vi "Agilent34410A VisaRW.vi"(0 "VISA Rsrc":refnum<visa-resource-name>="SR530", 1 "Timeout ms":u32=1000, 2 "EOS (Aucun)":string, 3 "Délais (0 ms)":u32, 5 "ChaineCom":string caption="Chaîne de commande", 7 "Nbcomm":i32=1 caption="Nombre de \nCommandes", 9 "Nbcaract":u32=100 caption="Nombre de \ncaractères à lire", 11 "error in (no error)":errorcluster, 12 "Lecture?(T)":bool=TRUE, 13 "Poll?(F)":bool) -> (4 "VISA Rsrc Out":refnum<visa-resource-name>="GPIB0::12::INSTR", 6 "ChaineRep":string caption="Chaîne de réponse", 8 "octet d'état":u16, 14 "Count out":u32=44 caption="Nombre de caractères lus", 15 "error out":errorcluster)   [LabVIEW 2019]
doc: "Ce VI envoie des commande d'écriture et de lecture VISA à l'appareil GPIB. Il permet de ne pas séparer un question de sa réponse. Pour que cela fonctionne toute lecture d'un instrument doit se faire par ce VI."
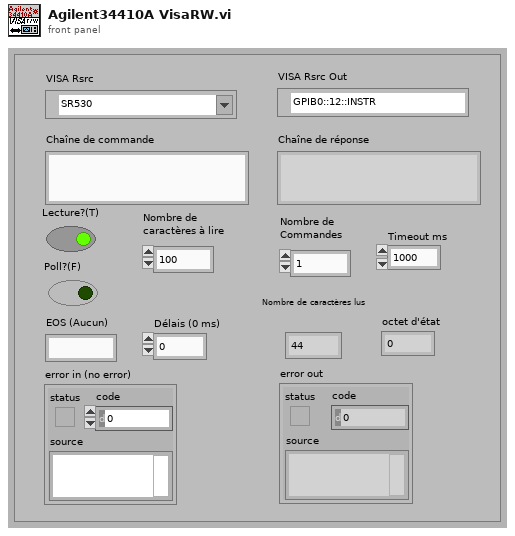
[diagram p1: front panel]
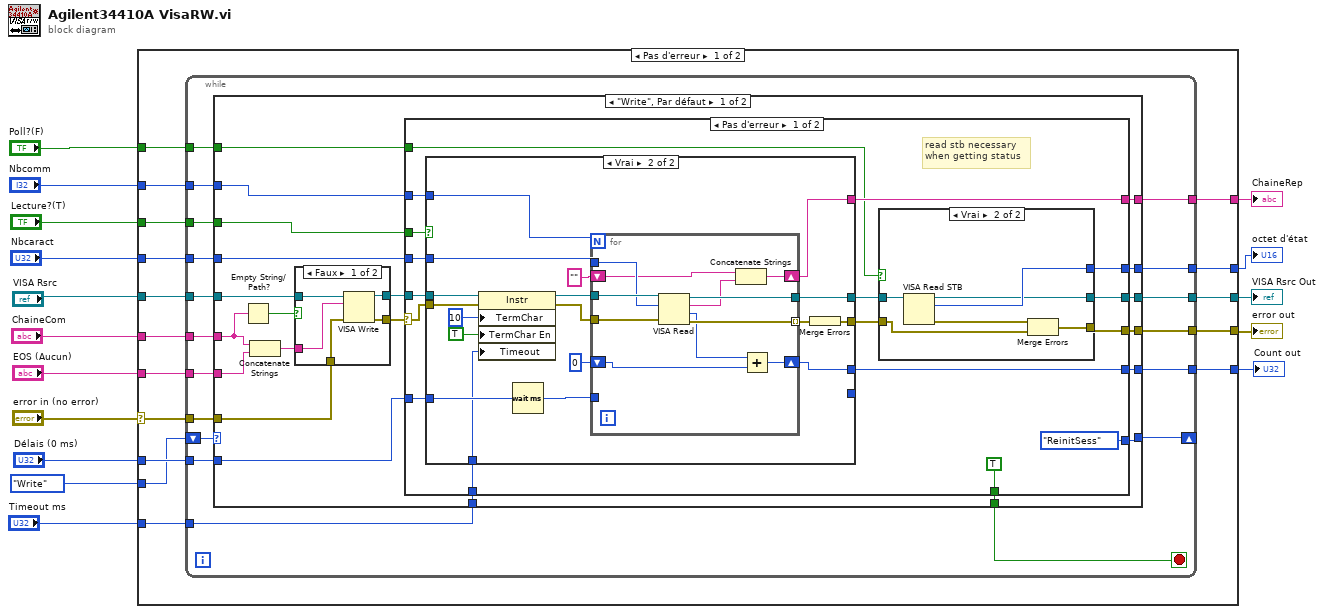
[diagram p0: block diagram]
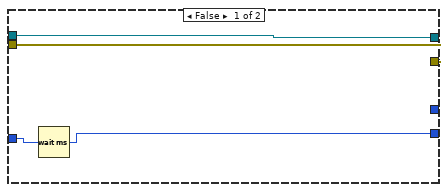
[diagram p3: hidden frame]
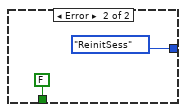
[diagram p4: hidden frame]
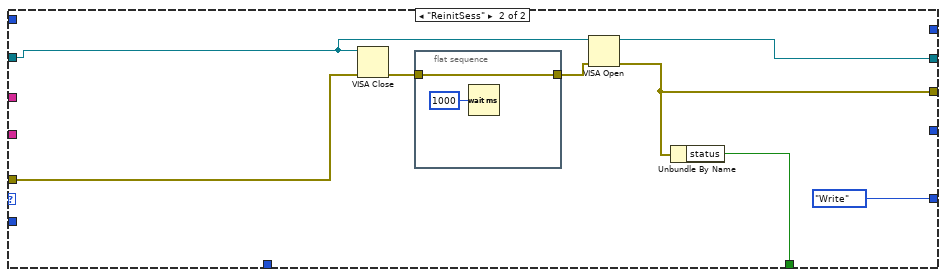
[diagram p6: hidden frame]
diagram:
  n1 = case shown="Pas d'erreur" "error in (no error)" {
    selector: "error in (no error)" -> [w30 w150]
    tunnel: "VISA Rsrc" -> [w31 w149]
    tunnel: [w21 w149] -> w9
    tunnel: "ChaineCom" -> [w23 _]
    tunnel: "EOS (Aucun)" -> [w32 _]
    tunnel: "Délais (0 ms)" -> [w29 _]
    tunnel: "Nbcaract" -> [w28 _]
    tunnel: "Lecture?(T)" -> [w27 _]
    tunnel: [w20 w150] -> w11
    tunnel: "Nbcomm" -> [w24 _]
    tunnel: [w26 _] -> w7
    tunnel: [w25 _] -> w6
    tunnel: "Poll?(F)" -> [w22 _]
    tunnel: [w19 _] -> w3
    tunnel: enum16{"Write", "ReinitSess"}."Write" -> [w18 _]
    tunnel: "Timeout ms" -> [w17 _]
    frame No Error {
      n2 = while {
        tunnel: w32 -> [w50]
        tunnel: w31 -> [w49]
        tunnel: w30 -> [w48]
        tunnel: w29 -> [w47]
        tunnel: w28 -> [w46]
        tunnel: w27 -> [w45]
        tunnel: [w44] -> w26
        tunnel: [w43] -> w25
        tunnel: w24 -> [w42]
        tunnel: w23 -> [w41]
        tunnel: w22 -> [w40]
        tunnel: [w39] -> w21
        tunnel: [w38] -> w20
        tunnel: [w37] -> w19
        shift-right: [w35] -> _
        shift-left: w18 -> [w36]
        tunnel: w17 -> [w33]
        stop <- w34 stop-if-true
        n3 = case shown="\"Write\", Par défaut" w36 {
          tunnel: w50 -> [w71 _]
          tunnel: w49 -> [w69 w145]
          tunnel: w48 -> [w68 w146]
          tunnel: w47 -> [w66 _]
          tunnel: w46 -> [w65 _]
          tunnel: w45 -> [w64 _]
          tunnel: [w63 _] -> w44
          tunnel: [w62 _] -> w43
          tunnel: w42 -> [w61 _]
          tunnel: w41 -> [w60 _]
          tunnel: w40 -> [w58 _]
          tunnel: [w57 w144] -> w39
          tunnel: [w56 w142] -> w38
          tunnel: [w55 _] -> w37
          tunnel: [w54 enum16{"Write", "ReinitSess"}."Write"] -> w35
          tunnel: [w52 w141] -> w34
          tunnel: w33 -> [w51 _]
          frame "Write", Default {
            n4 = Empty String/Path?(string/path=w60) -> (empty?=w59:bool)
            n5 = Concatenate Strings(w60, w71) -> (w70:string)
            n6 = case shown="Faux" w59 {
              tunnel: w70 -> [w136 _]
              tunnel: w69 -> [w135 w138]
              tunnel: w68 -> [w134 w137]
              tunnel: [w133 w138] -> w67
              tunnel: [w132 w137] -> w53
              frame False {
                n7 = VISA Write(VISA resource name=w135, write buffer=w136, error in (no error)=w134) -> (VISA resource name out=w133:refnum<visa-resource-name>, error out=w132:errorcluster)  [unwired: 1 out]
              }
              frame True {
              }
            }
            n8 = case shown="Pas d'erreur" w53 {
              selector: w53 -> [w74 _]
              tunnel: w67 -> [w88 _]
              tunnel: w66 -> [w87 _]
              tunnel: w65 -> [w86 _]
              tunnel: w64 -> [w85 _]
              tunnel: [w84 _] -> w63
              tunnel: [w83 _] -> w62
              tunnel: w61 -> [w82 _]
              tunnel: w58 -> [w81 _]
              tunnel: [w78 _] -> w57
              tunnel: [w77 _] -> w56
              tunnel: [w76 _] -> w55
              tunnel: [enum16{"Write", "ReinitSess"}."ReinitSess" enum16{"Write", "ReinitSess"}."ReinitSess"] -> w54
              tunnel: [TRUE FALSE] -> w52
              tunnel: w51 -> [w72 _]
              frame No Error {
                # "read stb necessary\nwhen getting status"
                n9 = case shown="Vrai" w85 {
                  tunnel: w88 -> [w100 w118]
                  tunnel: [w100 w103] -> w79
                  tunnel: w74 -> [w99 w107]
                  tunnel: [w99 w102] -> w80
                  tunnel: w86 -> [_ w116]
                  tunnel: w87 -> [w98 w115]
                  tunnel: w82 -> [_ w109]
                  tunnel: [_ w111] -> w84
                  tunnel: [_ w110] -> w83
                  tunnel: w72 -> [_ w101]
                  tunnel: [w97 _] -> _
                  frame False {
                    n10 = Wait (ms)(milliseconds to wait=w98) -> (millisecond timer value=w97:u32)
                  }
                  frame True {
                    n11 = property class="Instr"(reference=w118, error in=w107, "TermChar"=u8 10 ("Message Based Settings:Termination Character"), "TermChar En"=TRUE ("Message Based Settings:Termination Character Enable"), "Timeout"=w101) -> (reference out=w108:refnum<visa-resource-name>, error out=w106:errorcluster)
                    n12 = Wait (ms)(milliseconds to wait=w115) -> (millisecond timer value=w114:u32)
                    n13 = for {
                      N: w109 -> [_]
                      tunnel: w108 -> [w129]
                      tunnel: [w128] -> w103
                      tunnel: w106 -> [w127]
                      tunnel: [w126] -> w117 mode=indexing
                      tunnel: w116 -> [w125]
                      tunnel: w114 -> [_]
                      shift-right: [w123] -> w111
                      shift-left: "" -> [w122]
                      shift-right: [w120] -> w110
                      shift-left: u32 0 -> [w119]
                      n14 = VISA Read(VISA resource name=w129, byte count=w125, error in (no error)=w127) -> (VISA resource name out=w128:refnum<visa-resource-name>, read buffer=w124:string, return count=w121:u32, error out=w126:errorcluster)
                      n15 = Concatenate Strings(w122, w124) -> (w123:string)
                      n16 = Add(x=w121, y=w119) -> (x+y=w120:u32)
                    }
                    n17 = Merge Errors(w117) -> (w102:errorcluster)
                  }
                }
                n18 = case shown="Vrai" w81 {
                  tunnel: [w90 w91] -> w78
                  tunnel: [w89 w92] -> w77
                  tunnel: w80 -> [w89 w94]
                  tunnel: w79 -> [w90 w96]
                  tunnel: [_ w95] -> w76
                  frame False {
                  }
                  frame True {
                    n19 = VISA Read STB(11:w96) -> (0:w93:errorcluster, 2:w95:u16, 3:w91:refnum<visa-resource-name>)  [unwired: 1 in]
                    n20 = Merge Errors(w93, w94) -> (w92:errorcluster)
                  }
                }
              }
              frame Error {
              }
            }
          }
          frame "ReinitSess" {
            n21 = VISA Close(VISA resource name=w145, error in (no error)=w146) -> (error out=w139:errorcluster)
            n22 = flat-sequence {
              tunnel: [w147] -> w140
              tunnel: w139 -> [w147]
              frame #0 {
                n23 = Wait (ms)(milliseconds to wait=u32 1000) -> ()  [unwired: 1 out]
              }
            }
            n24 = VISA Open(error in (no error)=w140, VISA resource name=w145) -> (VISA resource name=w144:refnum<visa-resource-name>, error out=w142:errorcluster)  [unwired: 3 in]
            n25 = Unbundle By Name(w142) -> ("status"=w141:bool)
          }
        }
      }
    }
    frame Error {
    }
  }
  "error out" <- w11
  "VISA Rsrc Out" <- w9
  "ChaineRep" <- w7
  "Count out" <- w6
  "octet d'état" <- w3
